vi "calc CG.vi"(8 "error in (no error)":errorcluster) -> (0 "error out":errorcluster)   [LabVIEW 2023]
uses:
  ctrl defs/ctrl swerve module.ctl
  ctrl defs/ctrl XY coord.ctl
  Global INIT.vi
  Global odometry.vi
panel:
  out "x-y":T1[](array[typedef]) {"Y" format="%.4g"; "X" format="%.4g"}
  out "SWERVE INFO written to Global  odometry file":T2[](array[typedef])=[{"descr"="FR", "V"=0.0, "POS"=0.0, "target"=0.0, "ABS"=0.0, "from pivot to module"={"R"=0.0, "theta (deg)"=0.0, "theta spin (deg)"=0.0, "theta park (deg)"=0.0}, "coord wrt geom CTR"={"X"=12.214, "Y"=12.214}, "corner wt (lbm)"=18.4}, {"descr"="FL", "V"=0.0, "POS"=0.0, "target"=0.0, "ABS"=0.0, "from pivot to module"={"R"=0.0, "theta (deg)"=0.0, "theta spin (deg)"=0.0, "theta park (deg)"=0.0}, "coord wrt geom CTR"={"X"=-12.214, "Y"=12.214}, "corner wt (lbm)"=16.8}, {"descr"="RL", "V"=0.0, "POS"=0.0, "target"=0.0, "ABS"=0.0, "from pivot to module"={"R"=0.0, "theta (deg)"=0.0, "theta spin (deg)"=0.0, "theta park (deg)"=0.0}, "coord wrt geom CTR"={"X"=-12.214, "Y"=-12.214}, "corner wt (lbm)"=25.4}, {"descr"="RR", "V"=0.0, "POS"=0.0, "target"=0.0, "ABS"=0.0, "from pivot to module"={"R"=0.0, "theta (deg)"=0.0, "theta spin (deg)"=0.0, "theta park (deg)"=0.0}, "coord wrt geom CTR"={"X"=12.214, "Y"=-12.214}, "corner wt (lbm)"=22.8}] {"corner wt (lbm)" format="%#.3f"; "POS" format="%.3g"; "coord wrt geom CTR"."Y" format="%.4g"; "coord wrt geom CTR"."X" format="%.4g"; "from pivot to module"."theta park (deg)" format="%.4g"; "from pivot to module"."theta spin (deg)" format="%.4g"; "from pivot to module"."theta (deg)" format="%.4g"; "from pivot to module"."R" format="%.4g"; "ABS" format="%.3g"; "target" format="%.3g"; "V" format="%.3g"}
  out "coord wrt geom ctr":cluster{"X":dbl, "Y":dbl}[](array[cluster])=[{"X"=12.214, "Y"=12.214}, {"X"=-12.214, "Y"=12.214}, {"X"=-12.214, "Y"=-12.214}, {"X"=12.214, "Y"=-12.214}]
  out "CG XY":cluster{"X":dbl, "Y":dbl} {"X" format="%_3f"; "Y" format="%_3f"}
  out "wheel track & base":cluster{"X":dbl, "Y":dbl}={"X"=24.428, "Y"=24.428}
  out "weight (lbm)":dbl=104.0 format="%_4f"
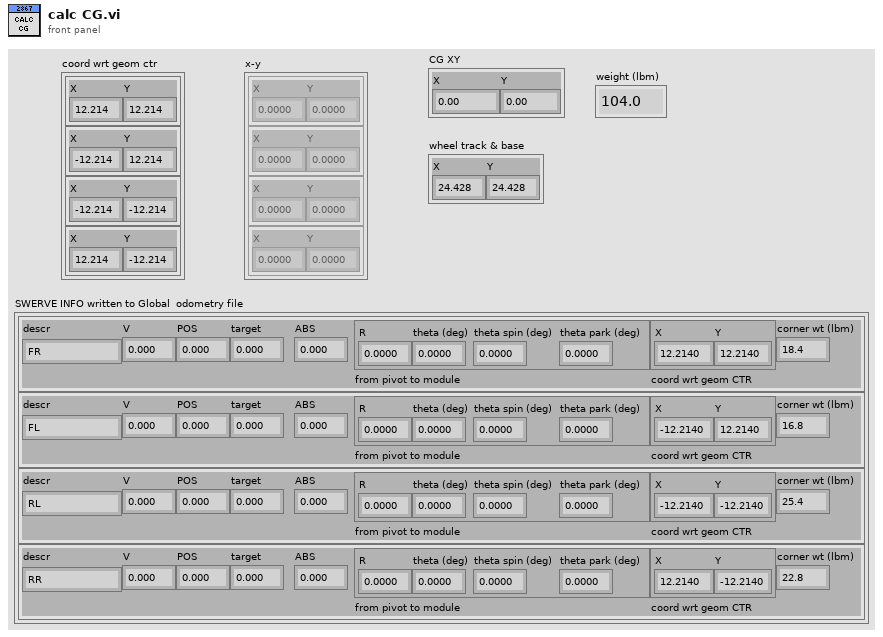
[diagram p1: front panel]
types:
  T1 = typedef "ctrl XY coord.ctl" = cluster{"X":dbl, "Y":dbl}
  T2 = typedef "ctrl swerve module.ctl" = cluster{"descr":string, "V":dbl, "POS":dbl, "target":dbl, "ABS":dbl, "from pivot to module":cluster{"R":dbl, "theta (deg)":dbl, "theta spin (deg)":dbl, "theta park (deg)":dbl}, "coord wrt geom CTR":cluster{"X":dbl, "Y":dbl}, "corner wt (lbm)":dbl}
  T3 = typedef "ctrl robot swerve dims.ctl" = cluster{"width":dbl, "depth":dbl}
  T4 = cluster{"description":string, "wrt geom CTR":cluster{"delX":i8, "delY":i8}}[]
  T5 = typedef "ctrl robot CG.ctl" = cluster{"mass (lbm)":dbl, "CG":T1, "Zcg":dbl}
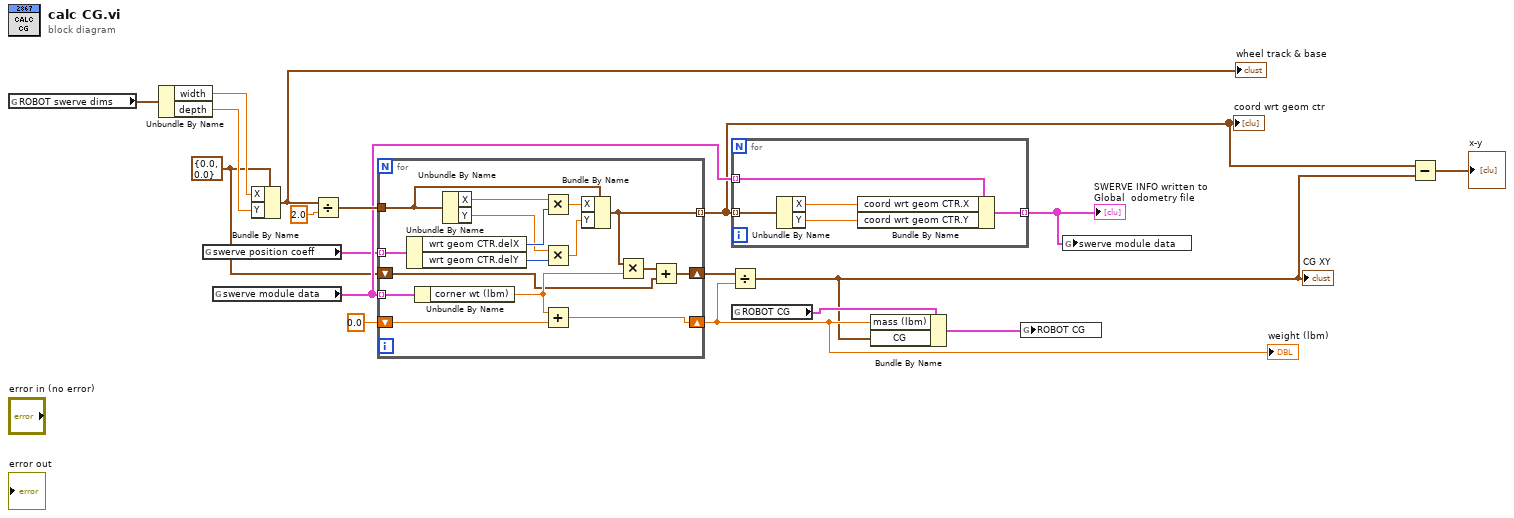
[diagram p0: block diagram]
diagram:
  w5 = T1 {"X"=0.0, "Y"=0.0} ("pivot center")
  n1 = global read "Global INIT.vi" "ROBOT swerve dims"() -> (w12:T3)
  n2 = Unbundle By Name(w12) -> ("width"=w16:dbl, "depth"=w15:dbl)
  n3 = global read "Global INIT.vi" "swerve position coeff"() -> (w4:T4)
  n4 = global read "Global odometry.vi" "swerve module data"() -> (w7:T2[])
  n5 = Bundle By Name(cluster=w5, "X"=w16, "Y"=w15) -> (w14:T1)
  "wheel track & base" <- w14
  n6 = Divide(x=w14, y=2.0) -> (x/y=w11:T1)
  n7 = for {
    tunnel: w11 -> [w34]
    tunnel: [w25] -> w3 mode=indexing
    tunnel: w7 -> [w31] mode=indexing
    shift-right: [w24] -> w9
    shift-left: 0.0 -> [w30]
    shift-right: [w21] -> w8
    shift-left: w5 -> [w20]
    tunnel: w4 -> [w19] mode=indexing
    n8 = Unbundle By Name(w19) -> ("wrt geom CTR.delX"=w29:i8, "wrt geom CTR.delY"=w26:i8)
    n9 = Unbundle By Name(w31) -> ("corner wt (lbm)"=w23:dbl)
    n10 = Unbundle By Name(w34) -> ("X"=w32:dbl, "Y"=w27:dbl)
    n11 = Multiply(x=w32, y=w29) -> (x*y=w33:dbl)
    n12 = Multiply(x=w27, y=w26) -> (x*y=w28:dbl)
    n13 = Add(x=w23, y=w30) -> (x+y=w24:dbl)
    n14 = Bundle By Name(cluster=w34, "X"=w33, "Y"=w28) -> (w25:T1)
    n15 = Multiply(x=w25, y=w23) -> (x*y=w22:T1)
    n16 = Add(x=w22, y=w20) -> (x+y=w21:T1)
  }
  "weight (lbm)" <- w9
  "coord wrt geom ctr" <- w3
  n17 = Divide(x=w8, y=w9) -> (x/y=w2:T1)
  "CG XY" <- w2
  n18 = for {
    tunnel: w7 -> [w39] mode=indexing
    tunnel: [w38] -> w6 mode=indexing
    tunnel: w3 -> [w37] mode=indexing
    n19 = Unbundle By Name(w37) -> ("X"=w36:dbl, "Y"=w35:dbl)
    n20 = Bundle By Name(cluster=w39, "coord wrt geom CTR.X"=w36, "coord wrt geom CTR.Y"=w35) -> (w38:T2)
  }
  "SWERVE INFO written to Global  odometry file" <- w6
  n21 = global read "Global INIT.vi" "ROBOT CG"() -> (w18:T5)
  n22 = Bundle By Name(cluster=w18, "mass (lbm)"=w9, "CG"=w2) -> (w17:T5)
  n23 = global write "Global INIT.vi" "ROBOT CG"(w17) -> ()
  n24 = global write "Global odometry.vi" "swerve module data"(w6) -> ()
  n25 = Subtract(x=w3, y=w2) -> (x-y=→"x-y":T1[])
